vi "subvi2.vi"(3 "Numeric":dbl) -> (1 "Numeric 4":dbl, 2 "Numeric 2":dbl)   [LabVIEW 2023]
panel:
  in  "Numeric 3":dbl
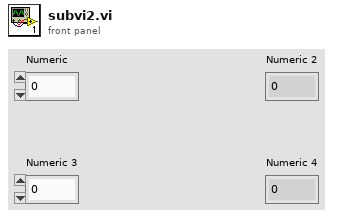
[diagram p1: front panel]
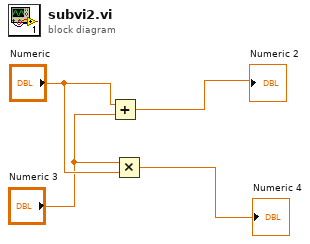
[diagram p0: block diagram]
diagram:
  n1 = Add(x="Numeric", y="Numeric 3") -> (x+y=→"Numeric 2":dbl)
  n2 = Multiply(x="Numeric 3", y="Numeric") -> (x*y=→"Numeric 4":dbl)
